vi "IsFieldType.vi"(8 "error in (no error)":errorcluster, 9 "Coordinate":T1, 10 "Type":T2, 11 "SnakeGame in":refnum<class "SnakeGame.lvclass">) -> (0 "error out":errorcluster, 2 "IsType?":bool, 3 "SnakeGame out":refnum<class "SnakeGame.lvclass">)   [LabVIEW 2019, in "RT_Game.lvlib" / "SnakeGame.lvclass"]
uses:
  SnakeGame.lvclass
  GridValue.ctl
  Engine/Coordinate.ctl
  SnakeGame.lvclass/SnakeGame.ctl
  <vilib>/Utility/error.llb/Error Cluster From Error Code.vi
  <vilib>/ErrorRing/Error Ring.xnode
  Engine/Engine.lvclass
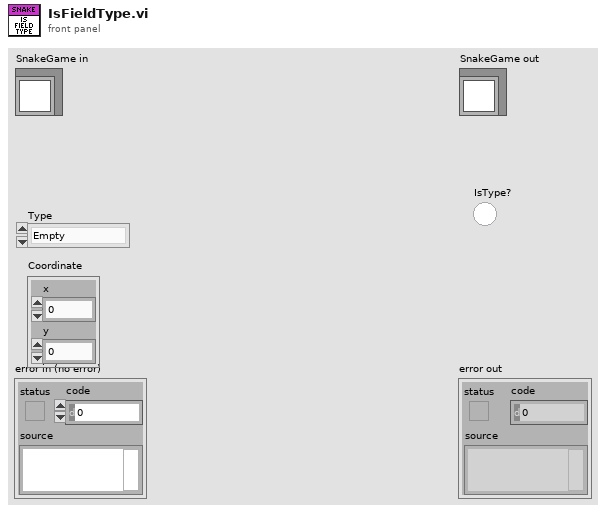
[diagram p1: front panel]
types:
  T1 = typedef "RT_Game.lvlib/Engine.lvclass/Coordinate.ctl" = cluster{"x":dbl, "y":dbl}
  T2 = typedef "RT_Game.lvlib/SnakeGame.lvclass/GridValue.ctl" = enum16{"Empty", "Snake1", "Snake1upLeft", "Snake1upRight", "Snake1downLeft", "Snake1downRight", "Snake2", "Snake2upLeft", "Snake2upRight", "Snake2downLeft", "Snake2downRight", "Score", "Speed", "Slow"}
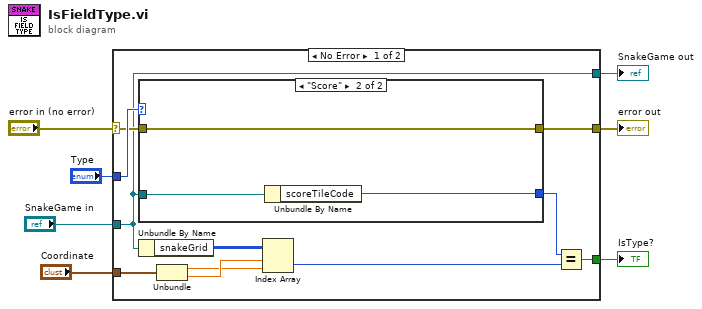
[diagram p0: block diagram]
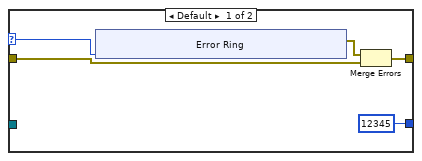
[diagram p2: hidden frame]
diagram:
  n1 = case shown="No Error" "error in (no error)" {
    selector: "error in (no error)" -> [w12 w35]
    tunnel: [w11 w35] -> w6
    tunnel: [w10 w34] -> w4
    tunnel: "SnakeGame in" -> [w10 w34]
    tunnel: "Coordinate" -> [w18 _]
    tunnel: "Type" -> [w13 _]
    tunnel: [w8 _] -> w1
    frame No Error {
      n2 = case shown="\"Score\"" w13 {
        selector: w13 -> [w23 _]
        tunnel: w10 -> [_ w33]
        tunnel: w12 -> [w22 w32]
        tunnel: [w21 w32] -> w11
        tunnel: [u32 12345 ("scoreTileCode") w31] -> w9
        frame Default {
          n3 = xnode "Error Ring"("parameter 0"=w23) -> ("error out"=w20:errorcluster)
          n4 = Merge Errors(w20, w22) -> (w21:errorcluster)
        }
        frame "Score" {
          n5 = Unbundle By Name(w33) -> ("scoreTileCode"=w31:u32)
        }
      }
      n6 = Unbundle By Name(w10) -> ("snakeGrid"=w16:u32[][])
      n7 = Unbundle(w18) -> ("x"=w15:dbl, "y"=w17:dbl)
      n8 = Index Array(array=w16, index (row)=w17, index (col)=w15) -> (element=w14:u32)
      n9 = Equal?(x=w9, y=w14) -> (x = y?=w8:bool)
    }
    frame Error {
    }
  }
  "error out" <- w6
  "SnakeGame out" <- w4
  "IsType?" <- w1
